vi "CheckMeasurementsSettings.vi"(8 "error in (no error)":errorcluster, 11 "NHRDCPower in":refnum<class "NHRDCPower.lvclass">) -> (0 "error out":errorcluster, 3 "NHRDCPower out":refnum<class "NHRDCPower.lvclass">)   [LabVIEW 2018, in "AcPwrPlugins.lvlib" / "NHRDCPower.lvclass"]
uses:
  NHRDCPower.lvclass
  <vilib>/Utility/error.llb/Error Cluster From Error Code.vi
  <vilib>/ErrorRing/Error Ring.xnode
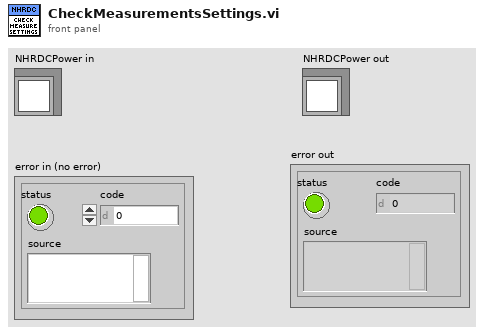
[diagram p1: front panel]
types:
  T1 = typedef "AcPwrPlugins.lvlib/NHRDCPower.lvclass/Device(s)Settings.ctl" = cluster{"Handle":string, "Name":string, "id query (Yes)":bool, "reset device (Yes)":bool, "Connected":bool, "Voltage Range (V)":dbl[], "Timing":cluster{"TimingOn":enum16{""}, "Hours":u32, "Minutes":u32, "Seconds":dbl, "CutoffVoltage":dbl}, "Initial Battery Detect Voltage (0)":sgl, "SafetySettings":cluster{"SetWatchDog":bool, "Voltage (V)":sgl, "Current (A)":sgl, "Power (W)":sgl, "Voltage Delay (s)":sgl, "Current Delay (s)":sgl, "Power Delay (s)":sgl}, "Options String":string, "Aperture Time (s)":sgl, "operating state (Off)":i32, "OutputSettings":cluster{"Voltage (V)":sgl, "Current (A)":sgl, "Resistance (Ohms)":sgl, "Power (W)":sgl, "Enable Voltage":bool, "Enable Current":bool, "Enable Resistance":bool, "Enable Power":bool, "Delay After (s)":sgl, "Wait Value (V, A, W)":sgl, "Enable Wait":bool, "Wait on Value":i32}[], "SlewRate":cluster{"Set Voltage Rate V/S":sgl, "Set Current Rate A/S":sgl, "Set Resistance Rate R/S":sgl, "Set Power Rate W/S":sgl}}[]
  T2 = typedef "AcPwrPlugins.lvlib/NHRDCPower.lvclass/Measurements.ctl" = cluster{"Handle":string, "Name":string, "Enabled":bool, "Measurement Value":sgl, "btnMeasFetch":bool, "Measurement Type":i32, "Fetch Method":i32, "Fetch Time (s)":sgl}[]
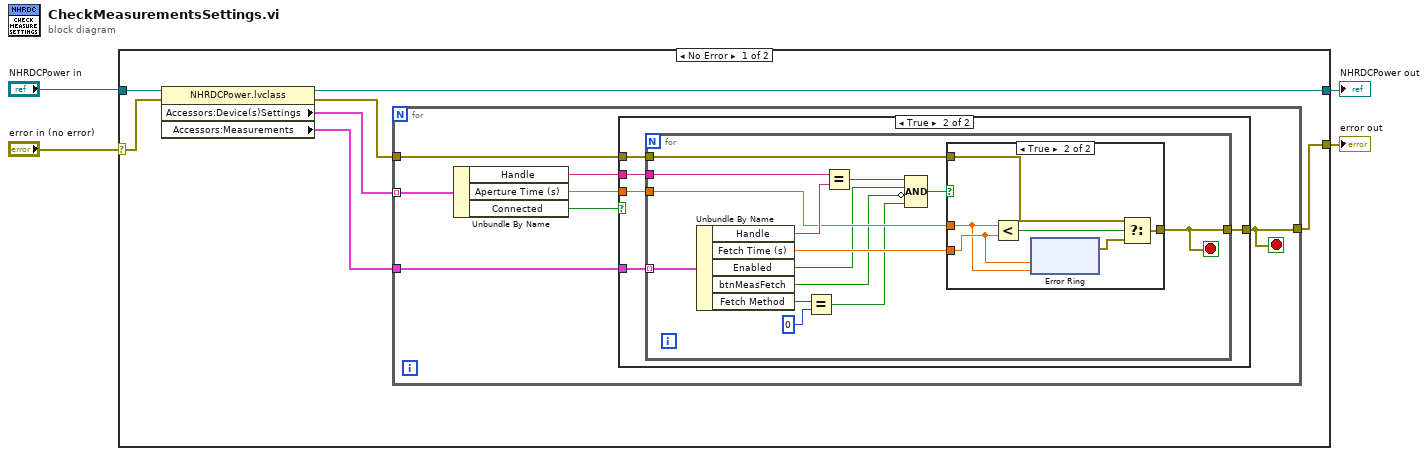
[diagram p0: block diagram]
diagram:
  n1 = case shown="No Error" "error in (no error)" {
    selector: "error in (no error)" -> [w10 w55]
    tunnel: [w5 w55] -> w1
    tunnel: [w11 w54] -> w2
    tunnel: "NHRDCPower in" -> [w9 w54]
    frame No Error {
      n2 = property class="NHRDCPower.lvclass"(reference=w9, error in=w10) -> (reference out=w11:refnum<class "NHRDCPower.lvclass">, error out=w6:errorcluster, "Accessors:Device(s)Settings"=w8:T1, "Accessors:Measurements"=w7:T2)
      n3 = for {
        tunnel: [w16] -> w5
        tunnel: w8 -> [w15] mode=indexing
        tunnel: w7 -> [w14]
        tunnel: w6 -> [w13]
        stop <- w16 stop-if-true
        n4 = Unbundle By Name(w15) -> ("Handle"=w18:string, "Aperture Time (s)"=w17:sgl, "Connected"=w12:bool)
        n5 = case shown="True" w12 {
          tunnel: w18 -> [_ w24]
          tunnel: w17 -> [_ w23]
          tunnel: [w19 w22] -> w16
          tunnel: w14 -> [_ w21]
          tunnel: w13 -> [w19 w20]
          frame False {
          }
          frame True {
            n6 = for {
              tunnel: w24 -> [w38]
              tunnel: w23 -> [w35]
              tunnel: [w27] -> w22
              tunnel: w21 -> [w26] mode=indexing
              tunnel: w20 -> [w25]
              stop <- w27 stop-if-true
              n7 = Unbundle By Name(w26) -> ("Handle"=w37:string, "Fetch Time (s)"=w34:sgl, "Enabled"=w32:bool, "btnMeasFetch"=w31:bool, "Fetch Method"=w30:i32)
              n8 = Equal?(x=w30, y=0) -> (x = y?=w28:bool)
              n9 = Equal?(x=w38, y=w37) -> (x = y?=w36:bool)
              n10 = Compound Arithmetic op=AND(w36, w32, invert w31, w28) -> (w33:bool)
              n11 = case shown="True" w33 {
                tunnel: w35 -> [_ w40]
                tunnel: w34 -> [_ w41]
                tunnel: [w39 w43] -> w27
                tunnel: w25 -> [w39 w42]
                frame False {
                }
                frame True {
                  n12 = Less?(x=w40, y=w41) -> (x < y?=w45:bool)
                  n13 = xnode "Error Ring"("parameter 0"=w41, "parameter 1"=w40) -> ("error out"=w44:errorcluster)
                  n14 = Select(t=w42, s=w45, f=w44) -> (s? t:f=w43:errorcluster)
                }
              }
            }
          }
        }
      }
    }
    frame Error {
    }
  }
  "error out" <- w1
  "NHRDCPower out" <- w2
